vi "Get Error Info.vi"(11 "Actor in":refnum<class "Actor.lvclass">) -> (2 "Error Info":T1)   [LabVIEW 2020, in "jettl.lvlib" / "Actor.lvlib" / "Actor.lvclass"]
uses:
  Actor.lvclass
  Error Info.ctl
  Actor.lvlib
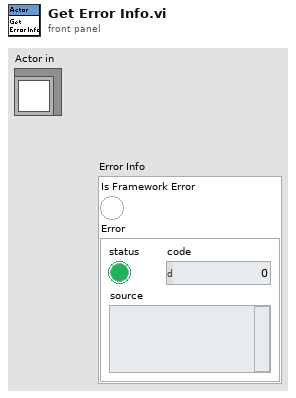
[diagram p1: front panel]
types:
  T1 = typedef "jettl.lvlib/Actor.lvlib/Error Info.ctl" = cluster{"Is Framework Error":bool, "Error":errorcluster}
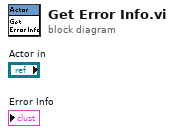
[diagram p0: block diagram]
diagram:
